vi "20170425-lecture4-1 write to spreadsheet.vi"() -> ()   [LabVIEW 2014]
uses:
  <vilib>/Utility/file.llb/Write To Spreadsheet File (DBL).vi
panel:
  out "Array":dbl[][](array[numeric])
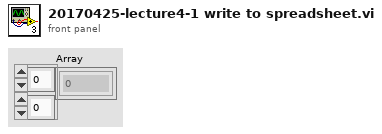
[diagram p1: front panel]
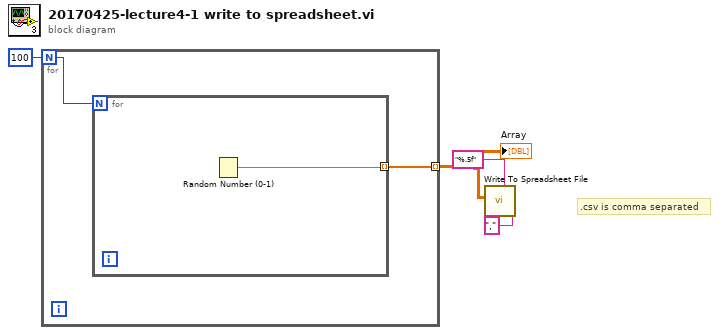
[diagram p0: block diagram]
diagram:
  # ".csv is comma separated"
  n1 = for {
    N: 100 -> [w6]
    tunnel: [w5] -> w3 mode=indexing
    n2 = for {
      N: w6 -> [_]
      tunnel: [w7] -> w5 mode=indexing
      n3 = Random Number (0-1)() -> (number: 0 to 1=w7:dbl)
    }
  }
  "Array" <- w3
  n4 = call-poly <vilib>:"Write To Spreadsheet File.vi"("delimiter (\\t)"="," ("delimiter (\\t)"), "format (%.3f)"="%.5f", "2D data"=w3) -> ()  [unwired: 5 in, 1 out]
